vi "Origin Column Set Get Data.vi"() -> ()   [LabVIEW 2020]
panel:
  out "Set Data B":errorcluster
  out "Set Data A":errorcluster
  out "Find Wks err":errorcluster
  out "get err C":errorcluster
  out "get err A":errorcluster
  out "get err B":errorcluster
  out "Basic Stats":string[][](table)
  # "This Example Shows how to access Origin Worksheet Columns\nA sample OPJ installed with Origin, which is also an Analysis Template to do simple basic statis computation, is used to demonstration the followings:\n\n1. Loading of an Origin OPJ file at a relative path from Origin installation\n2. Configuration of Worksheet Column objects, including to set them as Even Sampling (meaning no separate X column needed)\n3. Sending Data to columns in a sheet named \"Data\" and Getting data back from another sheet named \"Basic Stats\"\n4. Trigger to run Recalucate in Origin before getting data to show how Origin can be used as an Analysis Template"
  # "GetData Result"
  # "SetData Error Out"
  # "GetData Error Out"
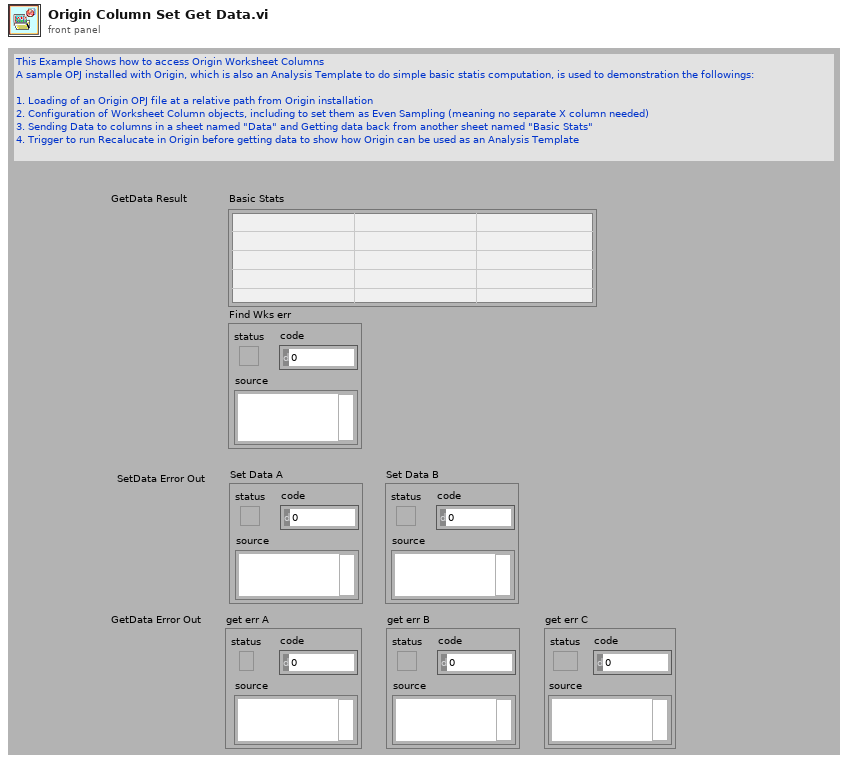
[diagram p1: front panel]
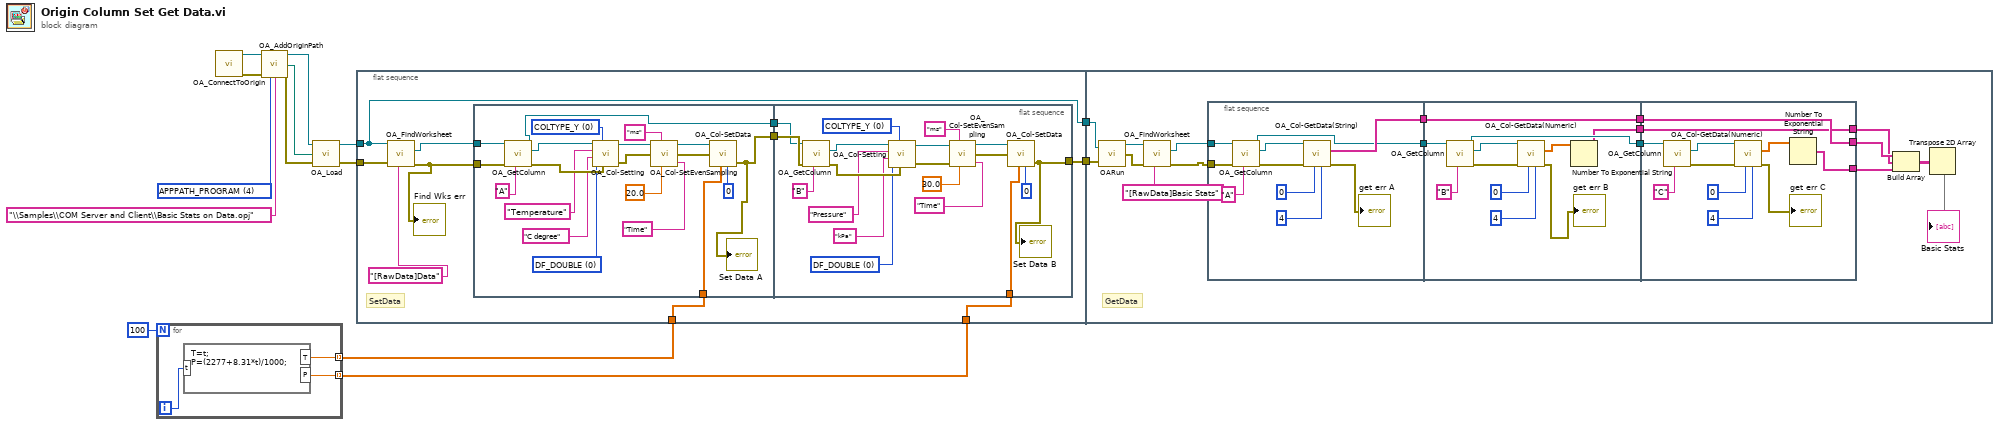
[diagram p0: block diagram]
diagram:
  w11 = 4 items=["APPPATH_USER"=2, "APPPATH_GROUP"=3, "APPPATH_PROGRAM"=4] ("Type")
  n1 = for {
    N: 100 -> [_]
    tunnel: [w16] -> w8 mode=indexing
    tunnel: [w15] -> w1 mode=indexing
    i -> [w17]
    n2 = formula code="T=t;\nP=(2277+8.31*t)/1000;"("t"=w17) -> ("T"=w16:dbl, "P"=w15:dbl)
  }
  n3 = call "OA_ConnectToOrigin.vi"() -> ("error out"=w4:errorcluster, "Origin.IOApplication"=w5:refnum<k7>)  [unwired: 8 in]
  n4 = call "OA_AddOriginPath.vi"("Origin.IOApplication"=w5, "error in (no error)"=w4, "Type"=w11, "Filename"="\\Samples\\COM Server and Client\\Basic Stats on Data.opj" ("related path")) -> ("Origin.IOApplication"=w14:refnum<k7>, "path out"=w12:path, "error out"=w13:errorcluster)  [unwired: 9 in]
  n5 = call "OA_Load.vi"("error in (no error)"=w13, "Path"=w12, "Origin.IOApplication"=w14) -> ("error out"=w6:errorcluster, "Origin.IOApplication"=w7:refnum<k7>)  [unwired: 1 out]
  n6 = flat-sequence {
    tunnel: w8 -> [w27]
    tunnel: w7 -> [w26]
    tunnel: [w26] -> w3
    tunnel: w6 -> [w25]
    tunnel: [w21] -> w2
    tunnel: w1 -> [w20]
    tunnel: w3 -> [w78]
    tunnel: w2 -> [w75]
    frame #0 {
      # "SetData"
      n7 = call "OA_FindWorksheet.vi"("Name"="[RawData]Data", "error in (no error)"=w25, "Origin.IOApplication"=w26) -> ("error out"=w19:errorcluster, "Origin.Worksheet"=w24:refnum<k7>)  [unwired: 6 in, 1 out]
      "Find Wks err" <- w19
      n8 = flat-sequence {
        tunnel: w24 -> [w47]
        tunnel: w19 -> [w46]
        tunnel: w27 -> [w41]
        tunnel: [w29] -> w22
        tunnel: [w33] -> w18
        tunnel: w22 -> [w55]
        tunnel: [w48] -> w21
        tunnel: w20 -> [w54]
        tunnel: w18 -> [w53]
        frame #0 {
          w30 = 0 items=["DF_NO_CHANGE"=-1, "DF_DOUBLE"=0, "DF_TEXT"=1, "DF_TIME"=2, "DF_DATE"=3, "DF_TEXT_NUMERIC"=9, "DF_FLOAT"=32, "DF_SHORT"=33, "DF_LONG"=34, "DF_CHAR"=35, "DF_BYTE"=38, "DF_USHORT"=39, "DF_ULONG"=40, "DF_COMPLEX"=41] ("DataFormat")
          w31 = 0 items=["COLTYPE_NO_CHANGE"=-1, "COLTYPE_Y"=0, "COLTYPE_NONE"=1, "COLTYPE_ERROR"=2, "COLTYPE_X"=3, "COLTYPE_LABEL"=4, "COLTYPE_Z"=5, "COLTYPE_X_ERROR"=6, "COLTYPE_GROUP"=7, "COLTYPE_SUBJECT"=8] ("Type")
          n9 = call "OA_GetColumn.vi"("Column Name/Index"="A", "error in (no error)"=w46, "Origin.Worksheet"=w47) -> ("error out"=w38:errorcluster, "Origin.Column"=w34:refnum<k7>, "Origin.Worksheet"=w33:refnum<k7>)  [unwired: 6 in]
          n10 = call "OA_Col-Setting.vi"("Origin.Column"=w34, "Type"=w31, "LongName"="Temperature", "Units"="C degree", "error in (no error)"=w38, "DataFormat"=w30) -> ("Origin.Column Out"=w39:refnum<k7>, "error out"=w35:errorcluster)  [unwired: 1 in]
          n11 = call "OA_Col-SetEvenSampling.vi"("Origin.Column"=w39, "Units"="ms", "error in (no error)"=w35, "XInc"=20.0, "LongName"="Time") -> ("Origin.Column Out"=w32:refnum<k7>, "error out"=w40:errorcluster)  [unwired: 1 in]
          n12 = call "OA_Col-SetData.vi"("Origin.Column"=w32, "error in (no error)"=w40, "data"=w41, "nOffset"=0) -> ("error out"=w29:errorcluster)  [unwired: 3 in, 2 out]
          "Set Data A" <- w29
        }
        frame #1 {
          w49 = 0 items=["DF_NO_CHANGE"=-1, "DF_DOUBLE"=0, "DF_TEXT"=1, "DF_TIME"=2, "DF_DATE"=3, "DF_TEXT_NUMERIC"=9, "DF_FLOAT"=32, "DF_SHORT"=33, "DF_LONG"=34, "DF_CHAR"=35, "DF_BYTE"=38, "DF_USHORT"=39, "DF_ULONG"=40, "DF_COMPLEX"=41] ("DataFormat")
          w50 = 0 items=["COLTYPE_NO_CHANGE"=-1, "COLTYPE_Y"=0, "COLTYPE_NONE"=1, "COLTYPE_ERROR"=2, "COLTYPE_X"=3, "COLTYPE_LABEL"=4, "COLTYPE_Z"=5, "COLTYPE_X_ERROR"=6, "COLTYPE_GROUP"=7, "COLTYPE_SUBJECT"=8] ("Type")
          n13 = call "OA_GetColumn.vi"("Column Name/Index"="B", "error in (no error)"=w55, "Origin.Worksheet"=w53) -> ("error out"=w59:errorcluster, "Origin.Column"=w52:refnum<k7>)  [unwired: 6 in, 1 out]
          n14 = call "OA_Col-Setting.vi"("Origin.Column"=w52, "Type"=w50, "LongName"="Pressure", "Units"="kPa", "error in (no error)"=w59, "DataFormat"=w49) -> ("Origin.Column Out"=w60:refnum<k7>, "error out"=w56:errorcluster)  [unwired: 1 in]
          n15 = call "OA_Col-SetEvenSampling.vi"("Origin.Column"=w60, "Units"="ms", "error in (no error)"=w56, "XInc"=30.0, "LongName"="Time") -> ("Origin.Column Out"=w51:refnum<k7>, "error out"=w61:errorcluster)  [unwired: 1 in]
          n16 = call "OA_Col-SetData.vi"("Origin.Column"=w51, "error in (no error)"=w61, "data"=w54, "nOffset"=0) -> ("error out"=w48:errorcluster)  [unwired: 3 in, 2 out]
          "Set Data B" <- w48
        }
      }
    }
    frame #1 {
      # "GetData"
      n17 = call "OARun.vi"("Origin.IOApplication"=w78, "Error IO"=w75) -> ("Origin.IOApplication"=w77:refnum<k7>, "Error IO Out"=w76:errorcluster)  [unwired: 1 out]
      n18 = call "OA_FindWorksheet.vi"("Name"="[RawData]Basic Stats", "error in (no error)"=w76, "Origin.IOApplication"=w77) -> ("error out"=w67:errorcluster, "Origin.Worksheet"=w82:refnum<k7>)  [unwired: 6 in, 1 out]
      n19 = flat-sequence {
        tunnel: w82 -> [w93]
        tunnel: w67 -> [w92]
        tunnel: [w88] -> w74
        tunnel: [w86] -> w72
        tunnel: w74 -> [w99]
        tunnel: [w99] -> w73
        tunnel: w72 -> [w98]
        tunnel: [w97] -> w71
        tunnel: [w95] -> w70
        tunnel: [w110] -> w81
        tunnel: w73 -> [w110]
        tunnel: w71 -> [w109]
        tunnel: w70 -> [w108]
        tunnel: [w108] -> w68
        tunnel: [w106] -> w69
        frame #0 {
          n20 = call "OA_GetColumn.vi"("Column Name/Index"="A", "error in (no error)"=w92, "Origin.Worksheet"=w93) -> ("error out"=w91:errorcluster, "Origin.Column"=w87:refnum<k7>, "Origin.Worksheet"=w86:refnum<k7>)  [unwired: 6 in]
          n21 = call "OA_Col-GetData(String).vi"("nEnd"=4, "nStart"=0, "error in (no error)"=w91, "Origin.Column"=w87) -> ("error out"=→"get err A":errorcluster, "data"=w88:string[])  [unwired: 5 in, 1 out]
        }
        frame #1 {
          n22 = call "OA_GetColumn.vi"("Column Name/Index"="B", "Origin.Worksheet"=w98) -> ("error out"=w103:errorcluster, "Origin.Column"=w100:refnum<k7>, "Origin.Worksheet"=w97:refnum<k7>)  [unwired: 7 in]
          n23 = call "OA_Col-GetData(Numeric).vi"("nEnd"=4, "nStart"=0, "error in (no error)"=w103, "Origin.Column"=w100) -> ("error out"=→"get err B":errorcluster, "data"=w96:dbl[])  [unwired: 5 in, 1 out]
          n24 = Number To Exponential String(number=w96) -> (E-format string=w95:string[])  [unwired: 3 in]
        }
        frame #2 {
          n25 = call "OA_GetColumn.vi"("Column Name/Index"="C", "Origin.Worksheet"=w109) -> ("error out"=w114:errorcluster, "Origin.Column"=w111:refnum<k7>)  [unwired: 7 in, 1 out]
          n26 = call "OA_Col-GetData(Numeric).vi"("nEnd"=4, "nStart"=0, "error in (no error)"=w114, "Origin.Column"=w111) -> ("error out"=→"get err C":errorcluster, "data"=w107:dbl[])  [unwired: 5 in, 1 out]
          n27 = Number To Exponential String(number=w107) -> (E-format string=w106:string[])  [unwired: 3 in]
        }
      }
      n28 = Build Array(w81, w68, w69) -> (w80:string[][])
      n29 = Transpose 2D Array(2D array=w80) -> (transposed array=→"Basic Stats":string[][])
    }
  }
